vi "Pruebas_dash.vi"() -> ()   [LabVIEW 2024]
panel:
  in  "Colors [4]":cluster{u32, u32}[](array[cluster])
  in  "Blank Button":bool caption="BATERIA"
  # "SAI PLANTA"
  # "Modo:"
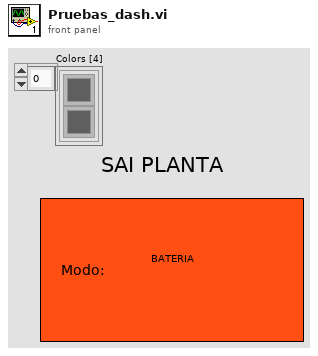
[diagram p1: front panel]
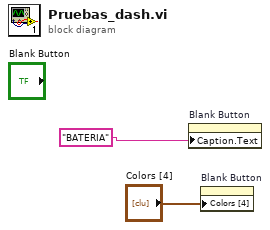
[diagram p0: block diagram]
diagram:
  n1 = property on="Blank Button" class="Bool"("Caption.Text"="BATERIA") -> ()  [unwired: 2 in, 2 out]
  n2 = property on="Blank Button" class="Bool"("Colors [4]"="Colors [4]") -> ()  [unwired: 2 in, 2 out]
